vi "Write reference clock source (Internal).vi"(8 "error in (no error)":errorcluster, 10 "reference clock source (Internal)":i32(ring) items=["Internal"=0, "External"=1, "RTSI Clock"=101], 11 "FgenPluginsBase in":refnum<class "FgenPluginsBase.lvclass">) -> (0 "error out":errorcluster, 3 "FgenPluginsBase out":refnum<class "FgenPluginsBase.lvclass">)   [LabVIEW 2018, in "FgenPlugins.lvlib" / "FgenPluginsBase.lvclass"]
uses:
  FgenPluginsBase.lvclass
  FgenPluginsBase.lvclass/FgenPluginsBase.ctl
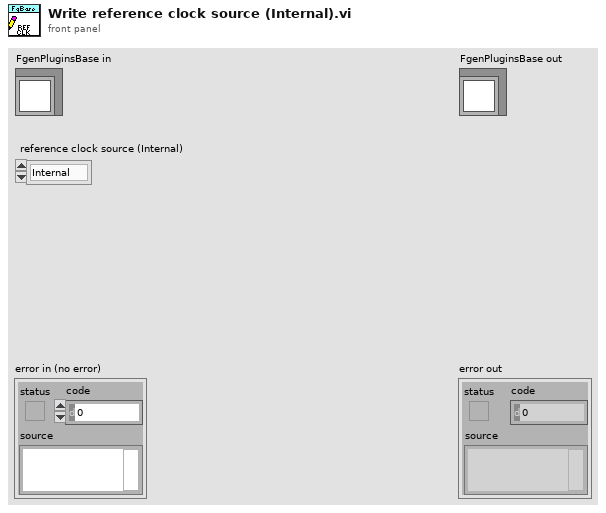
[diagram p1: front panel]
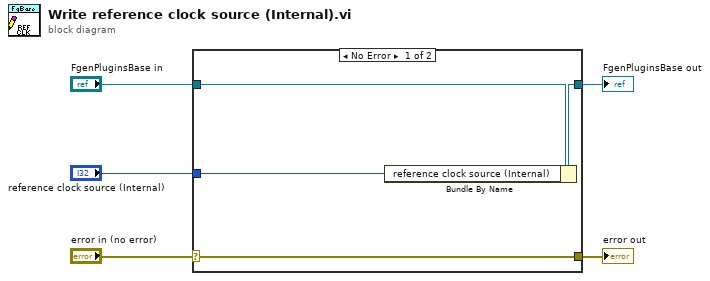
[diagram p0: block diagram]
diagram:
  n1 = case shown="No Error" "error in (no error)" {
    selector: "error in (no error)" -> [w9 w10]
    tunnel: [w9 w10] -> w4
    tunnel: [w7 w11] -> w2
    tunnel: "FgenPluginsBase in" -> [w8 w11]
    tunnel: "reference clock source (Internal)" -> [w6 _]
    frame No Error {
      n2 = Bundle By Name(cluster=w8, "reference clock source (Internal)"=w6) -> (w7:refnum<class "FgenPluginsBase.lvclass">)
    }
    frame Error {
    }
  }
  "error out" <- w4
  "FgenPluginsBase out" <- w2
